vi "test Loopback BC to RT.vi"(8 "error in":errorcluster, 11 "TestCase in":refnum<class "Loopback.lvclass">) -> (0 "error out":errorcluster, 3 "TestCase out":refnum<class "Loopback.lvclass">)   [LabVIEW 2020, in "Loopback.lvclass"]
uses:
  Loopback.lvclass
  C:/dev/niveristand-custom-device-testing-tools/VeriStandTestCase/VeriStandTestCase.lvclass
  <vilib>/numeric/Random Number (Range) U64.vi
  485b7c2b-8320-4722-9ec7-d01f27c65546.vi
  <vilib>/numeric/sub_Random U32.vi
  <vilib>/NI VeriStand/Execution/Workspace/NI VeriStand - Set Multiple Channel Values.vi
  <vilib>/NI VeriStand/Execution/Workspace/NI VeriStand - Get Multiple Channel Values.vi
  <vilib>/addons/_JKI Toolkits/VI Tester/TestCase.llb/TestCase.lvclass
  <vilib>/NI VeriStand/Execution/Workspace/NI_VS Workspace ExecutionAPI.lvlib
  0f9dda61-2c21-4955-8588-a8fc95227647.vi
  9a38d044-f7fa-4f05-ac83-bb7c785194b9.vi
  C:/Program Files (x86)/National Instruments/LabVIEW 2020/vi.lib/addons/_JKI Toolkits/VI Tester/TestCase.llb/TestCase.lvclass
  C:/dev/niveristand-ballard-milStd1553-custom-device/Source/Custom Device Support/Tests/System/Loopback/Loopback.lvclass
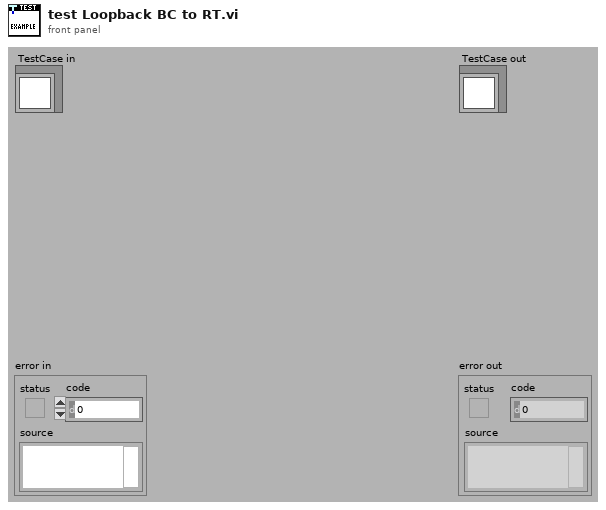
[diagram p1: front panel]
types:
  T1 = typedef "NI_VS Workspace ExecutionAPI.lvlib/WorkspaceAPI.ctl" = refnum<k24>
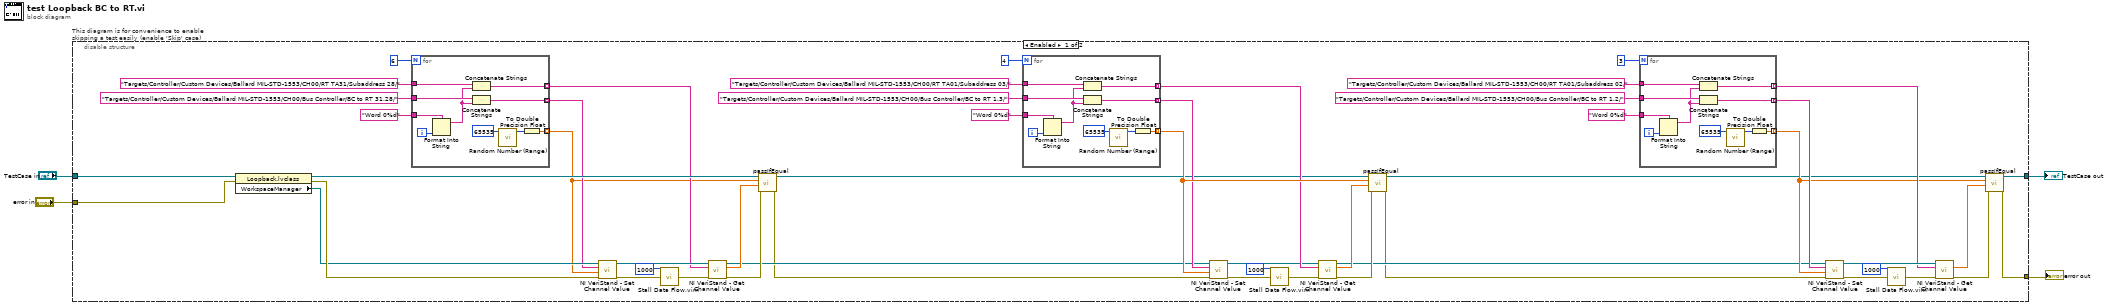
[diagram p0: block diagram]
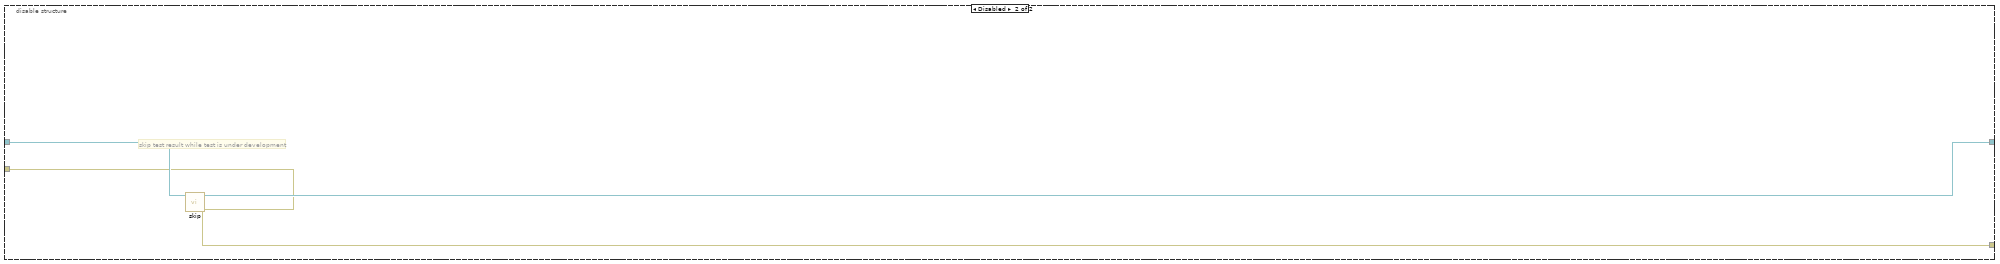
[diagram p2: hidden frame]
diagram:
  n1 = disable-structure "This diagram is for convenience to enable skipping a test easily (enable 'Skip' case)" shown="Enabled" {
    disable-tunnel: "TestCase in" -> [w47 w90]
    disable-tunnel: [w6 w88] -> w1
    disable-tunnel: [w5 w89] -> w3
    disable-tunnel: "error in" -> [w42 w87]
    frame Enabled {
      n2 = property class="Loopback.lvclass"(reference=w47, error in=w42) -> (reference out=w56:refnum<class "Loopback.lvclass">, error out=w51:errorcluster, "WorkspaceManager"=w49:T1)
      n3 = for {
        N: 6 -> [_]
        tunnel: "Targets/Controller/Custom Devices/Ballard MIL-STD-1553/CH00/Bus Controller/BC to RT 31.28/" ("Channel") -> [w85]
        tunnel: [w86] -> w45 mode=indexing
        tunnel: "Targets/Controller/Custom Devices/Ballard MIL-STD-1553/CH00/RT TA31/Subaddress 28/" ("Channel") -> [w84]
        tunnel: [w83] -> w43 mode=indexing
        tunnel: "Word 0%d" -> [w81]
        tunnel: [w77] -> w39 mode=indexing
        i -> [w82]
        n4 = Format Into String(format string=w81, w82) -> (resulting string=w80:string)  [unwired: 2 in, 1 out]
        n5 = Concatenate Strings(w84, w80) -> (w83:string)
        n6 = Concatenate Strings(w85, w80) -> (w86:string)
        n7 = call-poly <vilib>:"Random Number (Range).vi"("upper bound (100)"=u64 65535) -> ("number"=w79:u64)  [unwired: 10 in]
        n8 = To Double Precision Float(number=w79) -> (double precision float=w77:dbl)
      }
      n9 = call-poly <vilib>:"NI VeriStand - Set Channel Value.vi"("error in (no error)"=w51, "Values"=w39, "Channels"=w45, "WorkspaceManager in"=w49) -> ("error out"=w53:errorcluster, "WorkspaceManager out"=w55:T1)  [unwired: 6 in]
      n10 = call "Stall Data Flow.vim"("value in"=w53, "milliseconds to wait"=u32 1000) -> ("value out"=w54:errorcluster)  [unwired: 1 out]
      n11 = call-poly <vilib>:"NI VeriStand - Get Channel Value.vi"("error in (no error)"=w54, "Channels"=w43, "WorkspaceManager in"=w55) -> ("error out"=w50:errorcluster, "Values"=w48:dbl[], "WorkspaceManager out"=w24:T1)  [unwired: 6 in]
      n12 = call-dynamic "passIfEqual.vi"("error in (no error)"=w50, "y"=w48, "x"=w39, "TestCase in"=w56) -> ("error out"=w23:errorcluster, "TestCase out"=w25:refnum<class "Loopback.lvclass">)  [unwired: 6 in]
      n13 = for {
        N: 4 -> [_]
        tunnel: "Targets/Controller/Custom Devices/Ballard MIL-STD-1553/CH00/Bus Controller/BC to RT 1.3/" ("Channel") -> [w75]
        tunnel: [w76] -> w33 mode=indexing
        tunnel: "Targets/Controller/Custom Devices/Ballard MIL-STD-1553/CH00/RT TA01/Subaddress 03/" ("Channel") -> [w74]
        tunnel: [w73] -> w35 mode=indexing
        tunnel: "Word 0%d" -> [w71]
        tunnel: [w67] -> w38 mode=indexing
        i -> [w72]
        n14 = Format Into String(format string=w71, w72) -> (resulting string=w70:string)  [unwired: 2 in, 1 out]
        n15 = Concatenate Strings(w74, w70) -> (w73:string)
        n16 = Concatenate Strings(w75, w70) -> (w76:string)
        n17 = call-poly <vilib>:"Random Number (Range).vi"("upper bound (100)"=u64 65535) -> ("number"=w69:u64)  [unwired: 10 in]
        n18 = To Double Precision Float(number=w69) -> (double precision float=w67:dbl)
      }
      n19 = call-poly <vilib>:"NI VeriStand - Set Channel Value.vi"("error in (no error)"=w23, "Values"=w38, "Channels"=w33, "WorkspaceManager in"=w24) -> ("error out"=w28:errorcluster, "WorkspaceManager out"=w26:T1)  [unwired: 6 in]
      n20 = call "Stall Data Flow.vim"("value in"=w28, "milliseconds to wait"=u32 1000) -> ("value out"=w27:errorcluster)  [unwired: 1 out]
      n21 = call-poly <vilib>:"NI VeriStand - Get Channel Value.vi"("error in (no error)"=w27, "Channels"=w35, "WorkspaceManager in"=w26) -> ("error out"=w30:errorcluster, "Values"=w31:dbl[], "WorkspaceManager out"=w8:T1)  [unwired: 6 in]
      n22 = call-dynamic "passIfEqual.vi"("error in (no error)"=w30, "y"=w31, "x"=w38, "TestCase in"=w25) -> ("error out"=w7:errorcluster, "TestCase out"=w9:refnum<class "Loopback.lvclass">)  [unwired: 6 in]
      n23 = for {
        N: 3 -> [_]
        tunnel: "Targets/Controller/Custom Devices/Ballard MIL-STD-1553/CH00/Bus Controller/BC to RT 1.2/" ("Channel") -> [w65]
        tunnel: [w66] -> w15 mode=indexing
        tunnel: "Targets/Controller/Custom Devices/Ballard MIL-STD-1553/CH00/RT TA01/Subaddress 02/" ("Channel") -> [w64]
        tunnel: [w63] -> w13 mode=indexing
        tunnel: "Word 0%d" -> [w61]
        tunnel: [w57] -> w10 mode=indexing
        i -> [w62]
        n24 = Format Into String(format string=w61, w62) -> (resulting string=w60:string)  [unwired: 2 in, 1 out]
        n25 = Concatenate Strings(w64, w60) -> (w63:string)
        n26 = Concatenate Strings(w65, w60) -> (w66:string)
        n27 = call-poly <vilib>:"Random Number (Range).vi"("upper bound (100)"=u64 65535) -> ("number"=w59:u64)  [unwired: 10 in]
        n28 = To Double Precision Float(number=w59) -> (double precision float=w57:dbl)
      }
      n29 = call-poly <vilib>:"NI VeriStand - Set Channel Value.vi"("error in (no error)"=w7, "Values"=w10, "Channels"=w15, "WorkspaceManager in"=w8) -> ("error out"=w20:errorcluster, "WorkspaceManager out"=w22:T1)  [unwired: 6 in]
      n30 = call "Stall Data Flow.vim"("value in"=w20, "milliseconds to wait"=u32 1000) -> ("value out"=w21:errorcluster)  [unwired: 1 out]
      n31 = call-poly <vilib>:"NI VeriStand - Get Channel Value.vi"("error in (no error)"=w21, "Channels"=w13, "WorkspaceManager in"=w22) -> ("error out"=w18:errorcluster, "Values"=w17:dbl[])  [unwired: 6 in, 1 out]
      n32 = call-dynamic "passIfEqual.vi"("error in (no error)"=w18, "y"=w17, "x"=w10, "TestCase in"=w9) -> ("error out"=w5:errorcluster, "TestCase out"=w6:refnum<class "Loopback.lvclass">)  [unwired: 6 in]
    }
    frame Disabled {
      # "skip test result while test is under development"
      n33 = call <vilib>:"skip.vi"("error in (no error)"=w87, "TestCase in"=w90) -> ("error out"=w89:errorcluster, "TestCase out"=w88:refnum<class "Loopback.lvclass">)  [unwired: 8 in]
    }
  }
  "error out" <- w3
  "TestCase out" <- w1
